vi "Read Cyclinders.vi"(8 "error in (no error)":errorcluster, 11 "EST Knock Sensor in":refnum<class "Knock Sensor.lvclass">) -> (0 "error out":errorcluster, 2 "Cyclinders":u32, 3 "EST Knock Sensor out":refnum<class "Knock Sensor.lvclass">)   [LabVIEW 2015, in "Knock Sensor.lvclass"]
uses:
  Knock Sensor.lvclass
  Knock Sensor.lvclass/Knock Sensor.ctl
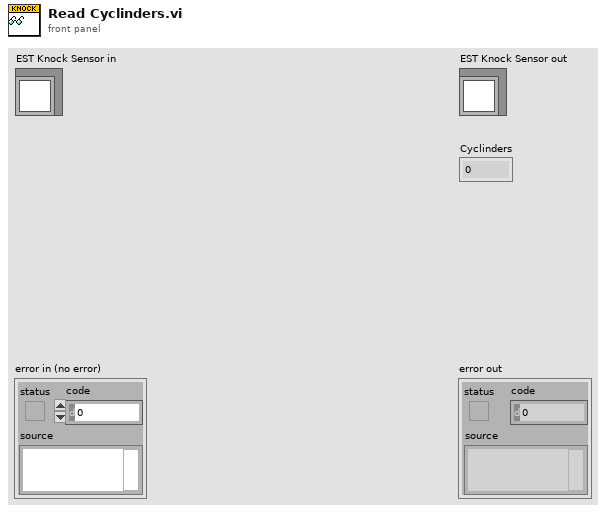
[diagram p1: front panel]
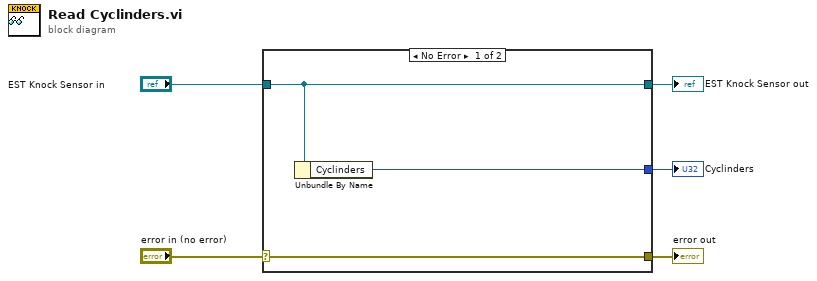
[diagram p0: block diagram]
diagram:
  n1 = case shown="No Error" "error in (no error)" {
    selector: "error in (no error)" -> [w8 w9]
    tunnel: [w8 w9] -> w4
    tunnel: [w7 w10] -> w2
    tunnel: "EST Knock Sensor in" -> [w7 w10]
    tunnel: [w6 _] -> w1
    frame No Error {
      n2 = Unbundle By Name(w7) -> ("Cyclinders"=w6:u32)
    }
    frame Error {
    }
  }
  "error out" <- w4
  "EST Knock Sensor out" <- w2
  "Cyclinders" <- w1
